vi "Essai.vi"() -> ()   [LabVIEW 2013, in "PDF Report.xctl"]
uses:
  PDF Report.xctl
panel:
  out "PDF Report 4":T21(xcontrol)
  in  "PDF Report 3":T21(xcontrol)
  out "PDF Report 2":T21(xcontrol)
  out "Path":path
  in  "PDF Report":T21(xcontrol)
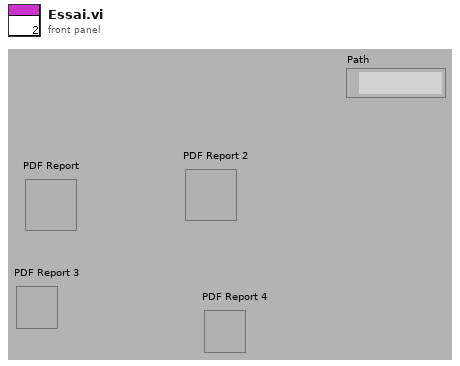
[diagram p1: front panel]
types:
  T1 = typedef "Font cluster.ctl" = cluster{"Name":string, "Size":T2, "Color":T3, "Style":cluster{"Bold":bool, "Italic":bool, "Underline":bool, "Strikeout":bool}}
  T2 = typedef "Font size.ctl" = sgl
  T3 = typedef "Font color.ctl" = u32
  T4 = typedef "Unit.ctl" = enum16{"inch", "mm"}
  T5 = typedef "Paragraphe cluster.ctl" = cluster{" Aligment":T6, "Line spacing":T7}
  T6 = typedef "Texte alignement.ctl" = enum16{"Select", "CENTER", "JUSTIFY", "LEFT", "RIGHT"}
  T7 = typedef "Line spacing.ctl" = enum16{"Select", "1.0", "1.5", "2.0"}
  T8 = typedef "Page dimensions.ctl" = cluster{"Start at page":i32, "Orientation":T9, "widht":sgl, "height":sgl, "Margin left":sgl, "Margin right":sgl, "Margin top":sgl, "Margin bottom":sgl}
  T9 = typedef "Page Orientation.ctl" = enum16{"Portrait", "Landscape"}
  T10 = typedef "Image or Table Caption.ctl" = cluster{"Caption":string, "Separator":string, "Position":enum16{"Above", "Below"}}
  T11 = typedef "Header Footer [ ].ctl" = T12[]
  T12 = typedef "Header Footer cluster.ctl" = cluster{"Start page":i32, "Type":T13, "Alignment":T14, "Vertical Alignement":T15, "Image (%)":sgl, "Page #":T16, "Text":string, "Path":string, "Font":T1, "Font refnum":refnum<k24>, "Line":cluster{"Line":T17, "Thickness (points)":sgl, "Colour":T3}}
  T13 = typedef "Header Footer Type.ctl" = enum16{"Select", "Text", "Text + hyperlink", "Page number", "Image", "Image + hyperlink"}
  T14 = typedef "Header footer horiz alignment.ctl" = enum16{"Left", "Center", "Right"}
  T15 = typedef "Cell Vertical alignment.ctl" = enum16{"TOP", "MIDDLE", "BOTTOM"}
  T16 = typedef "Page number.ctl" = cluster{"Text 1":string, "Text 2":string, "Text 3":string}
  T17 = typedef "Header Footer Line.ctl" = enum16{"No line", "Horizontal line"}
  T18 = typedef "Watermark cluster2.ctl" = cluster{"Show? (F)":bool, "Type":enum16{"Image", "Text"}, "Opacity (%)":sgl, "Rotate(°)":sgl, "Position":cluster{"Position":T19, "X":sgl, "Y":sgl}, "Image path":path, "Scaled(%)":sgl, "Image refnum":refnum<k24>, "Text":string, "Font":cluster{"Name":string, "Size":T2, "Color":T3}, "Font refnum":refnum<k24>, "Alignment":T14, "Automatic":bool}
  T19 = typedef "Watermark Position.ctl" = enum16{"Absolute", "Center (page)", "Center (text section)"}
  T20 = typedef "System Fonts.ctl" = cluster{"Font name [ ]":string[], "Font and file names [ ]":cluster{"Font name":string, "File name":string}[]}
  T21 = cluster{"Document":refnum<k24>, "Writer":refnum<k24>, "Default Font":refnum<k24>, "Default Font cluster":T1, "Path":path, "Unit (default = mm)":T4, "Paragraphe cluster":T5, "Pages dimensions [ ]":T8[], "Captions":cluster{"Image":T10, "Image counter":u16, "Table":T10, "Table counter":u16, "Font":T1}, "Header":T11, "Footer":T11, "Watermark ":T18, "Actual VI name":string, "System Fonts":T20}
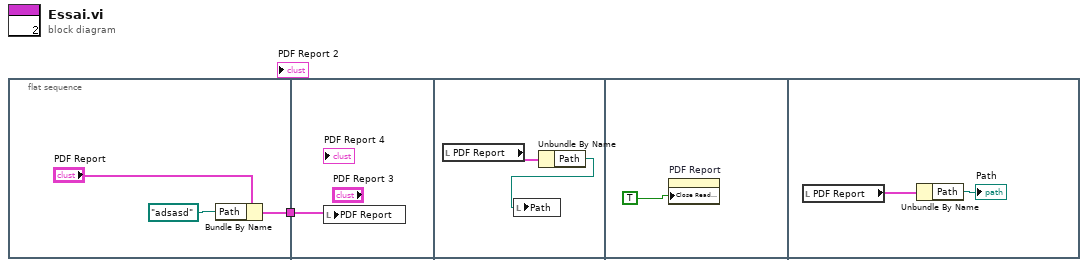
[diagram p0: block diagram]
diagram:
  n1 = flat-sequence {
    tunnel: [w2] -> w1
    tunnel: w1 -> [w5]
    frame #0 {
      n2 = Bundle By Name(cluster="PDF Report", "Path"=path "adsasd") -> (w2:T21)
    }
    frame #1 {
      n3 = local write "PDF Report"(w5) -> ()
    }
    frame #2 {
      n4 = local read "PDF Report"() -> (w7:T21)
      n5 = Unbundle By Name(w7) -> ("Path"=w6:path)
      n6 = local write "Path"(w6) -> ()
    }
    frame #3 {
      n7 = property on="PDF Report" class="PDF Report (strict)"("Close Reader and Writer refnum"=TRUE ("Clear")) -> ()  [unwired: 2 in, 2 out]
    }
    frame #4 {
      n8 = local read "PDF Report"() -> (w9:T21)
      n9 = Unbundle By Name(w9) -> ("Path"=→"Path":path)
    }
  }
